vi "make_axes_generic_grid.vi"(8 "length":sgl, 9 "Enum":enum16{"first", "second", "both"}(ring), 10 "Range":cluster{sgl, sgl}, 11 "Merged Array":T1(array[cluster])) -> (2 "Indices":u32[](array[numeric]), 3 "Vertex Array":cluster{"X":dbl, "Y":dbl, "x/y":dbl}[](array[cluster]))   [LabVIEW 2020, in "3DPC_SurfacePlot.xctl"]
uses:
  <vilib>/Native 3D Graph/xcontrol/3DPC_SurfacePlot.xctl
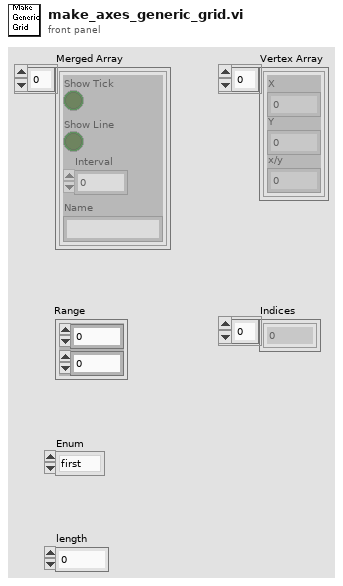
[diagram p1: front panel]
types:
  T1 = cluster{"Show Tick":bool, "Show Line":bool, "Interval":sgl, "Name":string}[]
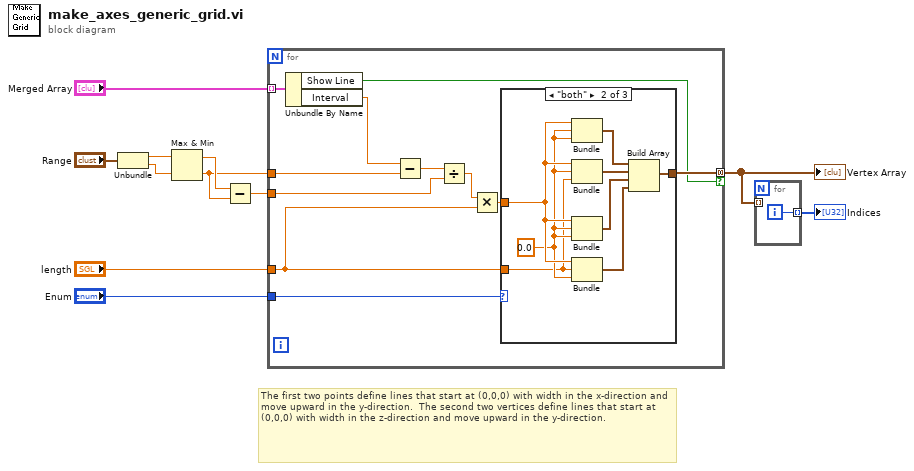
[diagram p0: block diagram]
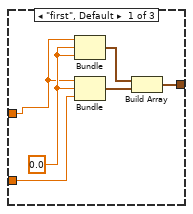
[diagram p2: hidden frame]
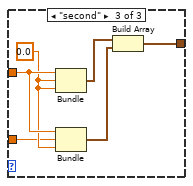
[diagram p3: hidden frame]
diagram:
  # "The first two points define lines that start at (0,0,0) with width in the x-direction and move upward in the y-direction.  The second two vertices define lines that start at (0,0,0) with width in the z-direction and move upward in the y-direction."
  n1 = Unbundle("Range") -> (w9:sgl, w8:sgl)
  n2 = Max & Min(x=w9, y=w8) -> (max(x,y)=w6:sgl, min(x,y)=w5:sgl)
  n3 = Subtract(x=w6, y=w5) -> (x-y=w4:sgl)
  n4 = for {
    tunnel: "Merged Array" -> [w22] mode=indexing
    tunnel: w5 -> [w20]
    tunnel: "length" -> [w15]
    tunnel: w4 -> [w18]
    tunnel: "Enum" -> [w14]
    tunnel: [w13] -> w1 mode=concatenating if=w12
    n5 = Unbundle By Name(w22) -> ("Show Line"=w12:bool, "Interval"=w21:sgl)
    n6 = Subtract(x=w21, y=w20) -> (x-y=w19:sgl)
    n7 = Divide(x=w19, y=w18) -> (x/y=w17:sgl)
    n8 = Multiply(x=w17, y=w15) -> (x*y=w16:sgl)
    n9 = case shown="\"both\"" w14 {
      tunnel: w16 -> [w25 w36 w42]
      tunnel: w15 -> [w24 w34 w40]
      tunnel: [w23 w31 w39] -> w13
      frame "first", Default {
        w28 = sgl 0.0 ("x*y")
        n10 = Bundle(w25, "x*y"=w28, "x*y"=w28) -> (w27:cluster{sgl, "x*y":sgl, "x*y":sgl})  [unwired: 1 out]
        n11 = Bundle(w25, "x*y"=w28, "length"=w24) -> (w26:cluster{sgl, "x*y":sgl, "length":sgl})  [unwired: 1 out]
        n12 = Build Array(w27, w26) -> (w23:cluster{sgl, "x*y":sgl, "length":sgl}[])
      }
      frame "both" {
        w35 = sgl 0.0 ("x*y")
        n13 = Bundle(w36, "x*y"=w35, "x*y"=w35) -> (w33:cluster{sgl, "x*y":sgl, "x*y":sgl})  [unwired: 1 out]
        n14 = Bundle(w36, "x*y"=w35, "length"=w34) -> (w32:cluster{sgl, "x*y":sgl, "length":sgl})  [unwired: 1 out]
        n15 = Bundle(w36, "x*y"=w35, "x*y"=w35) -> (w30:cluster{sgl, "x*y":sgl, "x*y":sgl})  [unwired: 1 out]
        n16 = Bundle(w36, "length"=w34, "x*y"=w35) -> (w29:cluster{sgl, "length":sgl, "x*y":sgl})  [unwired: 1 out]
        n17 = Build Array(w33, w32, w30, w29) -> (w31:cluster{sgl, "length":sgl, "x*y":sgl}[])
      }
      frame "second" {
        w41 = sgl 0.0 ("x*y")
        n18 = Bundle(w42, "x*y"=w41, "x*y"=w41) -> (w38:cluster{sgl, "x*y":sgl, "x*y":sgl})  [unwired: 1 out]
        n19 = Bundle(w42, "length"=w40, "x*y"=w41) -> (w37:cluster{sgl, "length":sgl, "x*y":sgl})  [unwired: 1 out]
        n20 = Build Array(w38, w37) -> (w39:cluster{sgl, "length":sgl, "x*y":sgl}[])
      }
    }
  }
  "Vertex Array" <- w1
  n21 = for {
    tunnel: w1 -> [_] mode=indexing
    tunnel: [w43] -> w3 mode=indexing
    i -> [w43]
  }
  "Indices" <- w3
